vi "RichToFlatni_bus_monitor_api_StreamBusReply.vi"(5 "OutputClusterType":T1, 11 "InputCluster":T7) -> (3 "OutputCluster":T1)   [LabVIEW 2025, in "bus_monitor_client.lvlib"]
uses:
  ni_bus_monitor_api_StreamBusReply.ctl
  ni_bus_monitor_api_CanCommState.ctl
  ni_bus_monitor_api_CommState.ctl
  ni_bus_monitor_api_LastCommError.ctl
  ni_bus_monitor_api_Frame.ctl
  ni_bus_monitor_api_ErrorInfo.ctl
  ni_bus_monitor_api_StreamBusReply_Flat.ctl
  ni_bus_monitor_api_CanCommState_Flat.ctl
  ni_bus_monitor_api_Frame_Flat.ctl
  ni_bus_monitor_api_ErrorInfo_Flat.ctl
  bus_monitor_client.lvlib
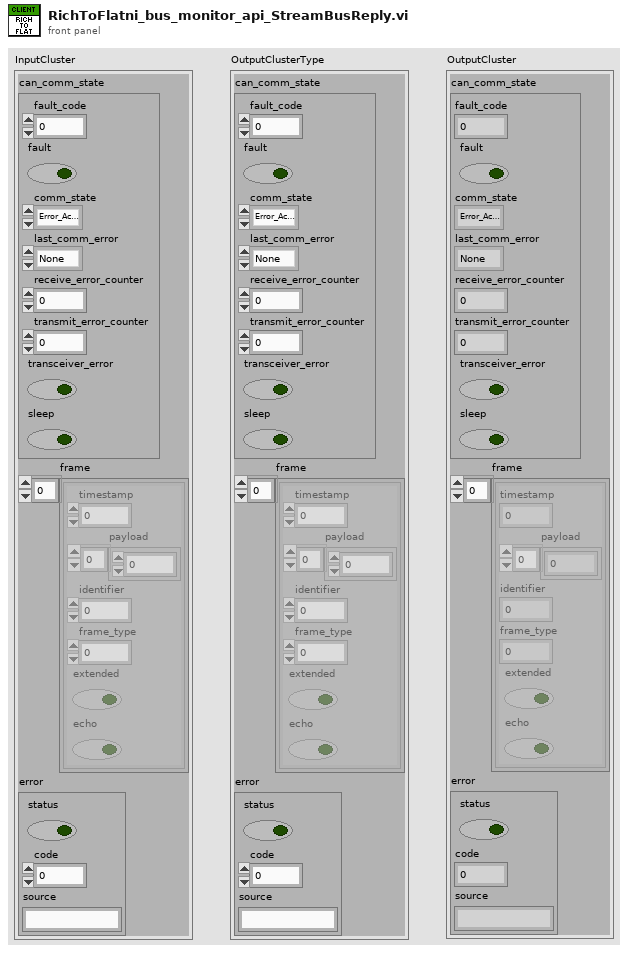
[diagram p1: front panel]
types:
  T1 = typedef "bus_monitor_client.lvlib/ni_bus_monitor_api_StreamBusReply_Flat.ctl" = cluster{"can_comm_state":T2, "frame":T5[], "error":T6}
  T2 = typedef "bus_monitor_client.lvlib/ni_bus_monitor_api_CanCommState_Flat.ctl" = cluster{"fault_code":i32, "fault":bool, "comm_state":T3, "last_comm_error":T4, "receive_error_counter":u32, "transmit_error_counter":u32, "transceiver_error":bool, "sleep":bool}
  T3 = typedef "bus_monitor_client.lvlib/ni_bus_monitor_api_CommState.ctl" = enum32{"Error_Active", "Error_Passive", "Bus_Off", "Init"}
  T4 = typedef "bus_monitor_client.lvlib/ni_bus_monitor_api_LastCommError.ctl" = enum32{"None", "Stuff", "Form", "ACK", "Bit1", "Bit0", "CRC"}
  T5 = typedef "bus_monitor_client.lvlib/ni_bus_monitor_api_Frame_Flat.ctl" = cluster{"timestamp":dbl, "payload":u8[], "identifier":u32, "frame_type":u32, "extended":bool, "echo":bool}
  T6 = typedef "bus_monitor_client.lvlib/ni_bus_monitor_api_ErrorInfo_Flat.ctl" = errorcluster
  T7 = typedef "bus_monitor_client.lvlib/ni_bus_monitor_api_StreamBusReply.ctl" = cluster{"can_comm_state":T8, "frame":T9[], "error":T10}
  T8 = typedef "bus_monitor_client.lvlib/ni_bus_monitor_api_CanCommState.ctl" = cluster{"fault_code":i32, "fault":bool, "comm_state":T3, "last_comm_error":T4, "receive_error_counter":u32, "transmit_error_counter":u32, "transceiver_error":bool, "sleep":bool}
  T9 = typedef "bus_monitor_client.lvlib/ni_bus_monitor_api_Frame.ctl" = cluster{"timestamp":dbl, "payload":u8[], "identifier":u32, "frame_type":u32, "extended":bool, "echo":bool}
  T10 = typedef "bus_monitor_client.lvlib/ni_bus_monitor_api_ErrorInfo.ctl" = errorcluster
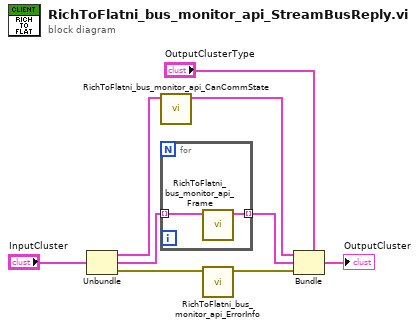
[diagram p0: block diagram]
diagram:
  n1 = Unbundle "Unbundle"("InputCluster") -> ("can_comm_state"=w6:T8, "frame"=w4:T9[], "error"=w2:T10)
  n2 = call "RichToFlatni_bus_monitor_api_CanCommState.vi"("InputCluster"=w6) -> ("OutputCluster"=w5:T2)  [unwired: 10 in]
  n3 = for {
    tunnel: w4 -> [w11] mode=indexing
    tunnel: [w10] -> w3 mode=indexing
    n4 = call "RichToFlatni_bus_monitor_api_Frame.vi"("InputCluster"=w11) -> ("OutputCluster"=w10:T5)  [unwired: 10 in]
  }
  n5 = call "RichToFlatni_bus_monitor_api_ErrorInfo.vi"("InputCluster"=w2) -> ("OutputCluster"=w1:T6)  [unwired: 10 in]
  n6 = Bundle "Bundle"(cluster="OutputClusterType", "can_comm_state"=w5, "frame"=w3, "error"=w1) -> (→"OutputCluster":T1)
